vi "Skip.vi"(7 "Description":string, 8 "error in (no error)":errorcluster, 9 "Message":string, 11 "LUnit Test Case In":refnum<class "LUnit Test Case.lvclass">) -> (0 "error out":errorcluster, 3 "LUnit Test Case Out":refnum<class "LUnit Test Case.lvclass">)   [LabVIEW 2020, in "LUnit Test Case.lvclass"]
doc: "Ignores results from the calling test method when evaluating the test case result. A description and message may be provided."
uses:
  LUnit Test Case.lvclass
  Core/Result/Type.ctl
  Core/Result/Result.ctl
  Core/Result/Status.ctl
  LUnit Test Case.lvclass/LUnit Test Case.ctl
  Core/Result/Result.lvlib
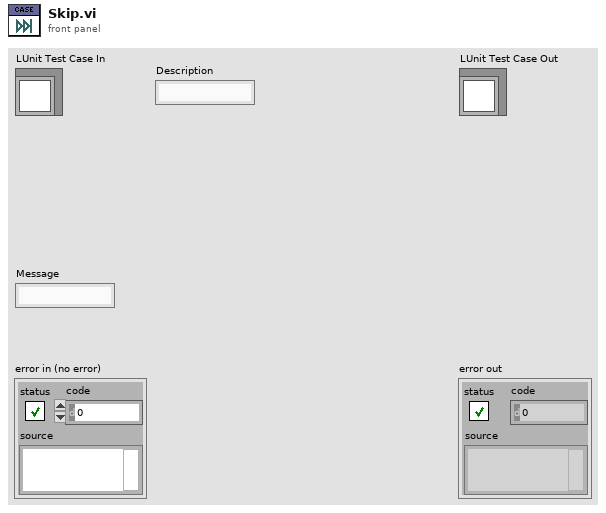
[diagram p1: front panel]
types:
  T1 = typedef "Result.lvlib/Type.ctl" = enum16{"Method", "Case", "Suite", "Pass", "Fail", "Skip", "Pass if", "Fail if", "Pass if Error", "Fail if Error", "Pass if Equal", "Fail if Equal"}
  T2 = typedef "Result.lvlib/Result.ctl" = cluster{"Name":string, "Message":string, "Description":string, "Status":T3, "Result Type":T1, "Execution Time":dbl}
  T3 = typedef "Result.lvlib/Status.ctl" = enum16{"", "Passed", "Failed", "Error", "Skipped", "Setup Error", "Broken", "Teardown Error"}
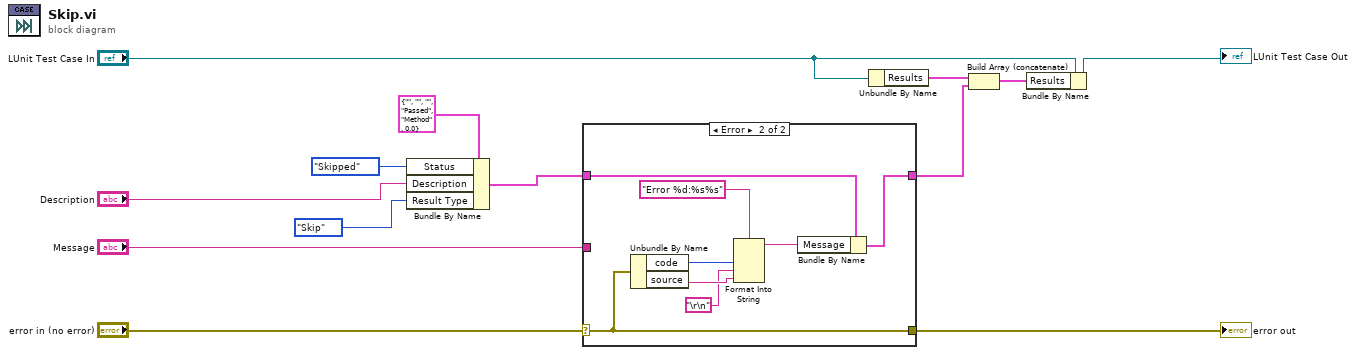
[diagram p0: block diagram]
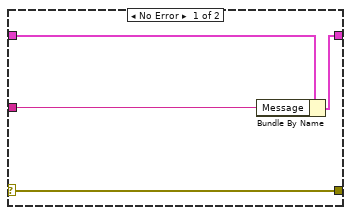
[diagram p2: hidden frame]
diagram:
  n1 = Bundle By Name(cluster=T2 {"Name"="", "Message"="", "Description"="", "Status"=enum."Passed", "Result Type"=enum."Method", "Execution Time"=0.0} ("Temporary Assertion Result"), "Status"=Status."Skipped", "Description"="Description", "Result Type"=Type."Skip") -> (w8:T2)
  n2 = case shown="Error" "error in (no error)" {
    selector: "error in (no error)" -> [w17 w24]
    tunnel: [w17 w24] -> w13
    tunnel: [w15 w25] -> w1
    tunnel: "Message" -> [w16 _]
    tunnel: w8 -> [w14 w18]
    frame No Error {
      n3 = Bundle By Name(cluster=w14, "Message"=w16) -> (w15:T2)
    }
    frame Error {
      n4 = Unbundle By Name(w24) -> ("code"=w22:i32, "source"=w20:string)
      n5 = Format Into String(format string="Error %d:%s%s", w22, "\r\n", w20) -> (resulting string=w21:string)  [unwired: 2 in, 1 out]
      n6 = Bundle By Name(cluster=w18, "Message"=w21) -> (w25:T2)
    }
  }
  "error out" <- w13
  n7 = Unbundle By Name("LUnit Test Case In") -> ("Results"=w4:T2[])
  n8 = Build Array (concatenate)(w4, w1) -> (w2:T2[])
  n9 = Bundle By Name(cluster="LUnit Test Case In", "Results"=w2) -> (→"LUnit Test Case Out":refnum<class "LUnit Test Case.lvclass">)
